vi "1820_IPS_to_DSC.vi"(0 "str":string[](array[string])=["CLMP"], 1 "str var":refnum<k21>[](array[refnum])=["ni.var.psp://housesoftheholy/MNK_18T/1820_IPS_Status", "ni.var.psp://housesoftheholy/MNK_18T/1820_IPS_Switch"], 2 "dbl":dbl[](array[numeric])=[0.0, -0.0, 0.0, 0.91, -0.0002, -0.0003, 81.9328, 94.8099], 3 "dbl var":refnum<k21>[](array[refnum])=["ni.var.psp://housesoftheholy/MNK_18T/1820_IPS_Magnet_Field", "ni.var.psp://housesoftheholy/MNK_18T/1820_IPS_PS_Field", "ni.var.psp://housesoftheholy/MNK_18T/1820_IPS_Target_Field", "ni.var.psp://housesoftheholy/MNK_18T/1820_IPS_Target_Field_Rate", "ni.var.psp://housesoftheholy/MNK_18T/1820_IPS_Voltage", "ni.var.psp://housesoftheholy/MNK_18T/1820_IPS_Current", "ni.var.psp://housesoftheholy/MNK_18T/1820_IPS_Level_N2", "ni.var.psp://housesoftheholy/MNK_18T/1820_IPS_Level_He", "ni.var.psp://housesoftheholy/MNK_18T/1820_IPS_Magnet_Temperature", "ni.var.psp://housesoftheholy/MNK_18T/1820_IPS_Magnet_Temperature_R", "ni.var.psp://housesoftheholy/MNK_18T/1820_IPS_M1_Current", "ni.var.psp://housesoftheholy/MNK_18T/1820_IPS_M1_Voltage", "ni.var.psp://housesoftheholy/MNK_18T/1820_IPS_M2_Current", "ni.var.psp://housesoftheholy/MNK_18T/1820_IPS_M2_Voltage", "ni.var.psp://housesoftheholy/MNK_18T/1820_IPS_M3_Current", "ni.var.psp://housesoftheholy/MNK_18T/1820_IPS_M3_Voltage"]) -> ()   [LabVIEW 2016, in "Instrument.OxfordVRM.lvclass"]
uses:
  Instrument.OxfordVRM.lvclass
panel:
  # "1820 IPS to DSC"
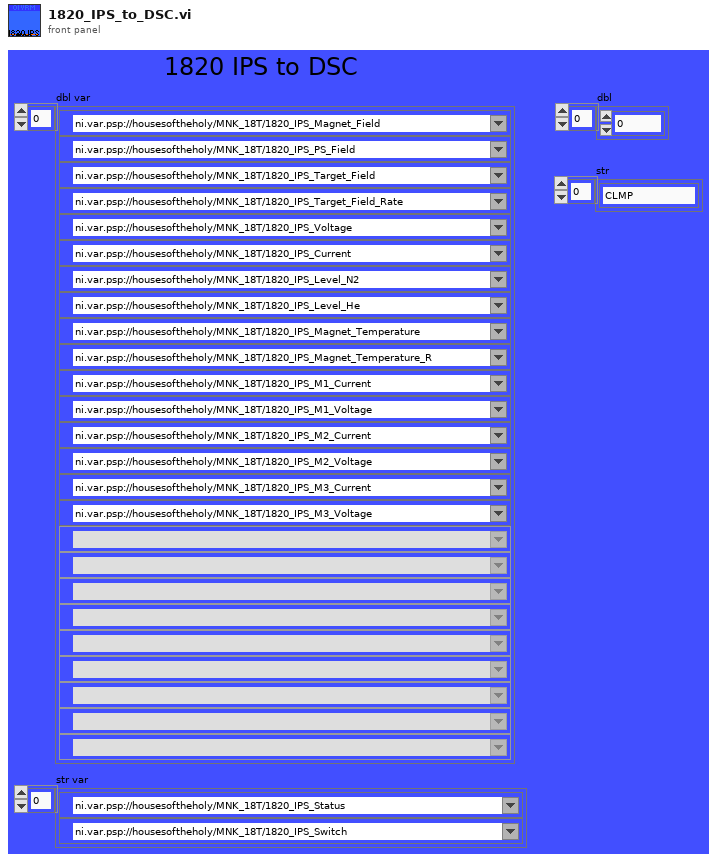
[diagram p1: front panel]
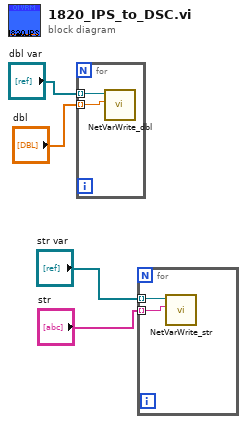
[diagram p0: block diagram]
diagram:
  n1 = for {
    tunnel: "dbl var" -> [w6] mode=indexing
    tunnel: "dbl" -> [w5] mode=indexing
    n2 = call "NetVarWrite_dbl.vi"("Numeric"=w5, "Refnum in"=w6) -> ()  [unwired: 9 in, 1 out]
  }
  n3 = for {
    tunnel: "str var" -> [w8] mode=indexing
    tunnel: "str" -> [w7] mode=indexing
    n4 = call "NetVarWrite_str.vi"("String"=w7, "Refnum in"=w8) -> ()  [unwired: 9 in, 1 out]
  }
